vi "Module Loop.vi"(8 "error in (no error)":errorcluster, 11 "Data Processor Module in":refnum<class "Data Processor Module.lvclass">) -> (0 "error out":errorcluster, 3 "Data Processor Module out":refnum<class "Data Processor Module.lvclass">)   [LabVIEW 2020, in "VolatusData.lvlib" / "Data Processor Module.lvclass"]
uses:
  Data Processor Module.lvclass
  C:/dev/lv20CE/relink/lv-volatus/Volatus/Module/Module.lvclass
  Volatus/Module/Module.lvclass
  New Data.ctl
  Volatus/Module/Module.lvclass/Module.ctl
  <vilib>/Utility/error.llb/Error Cluster From Error Code.vi
  Data Processor Module.lvclass/Data Processor Module.ctl
  VolatusData.lvlib
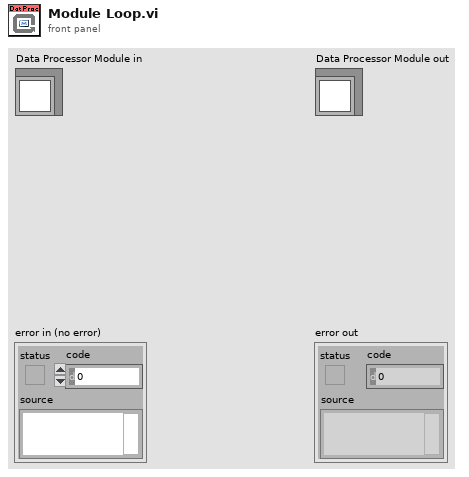
[diagram p1: front panel]
types:
  T1 = typedef "VolatusData.lvlib/New Data.ctl" = cluster{"Channels":waveform(dbl)[]}
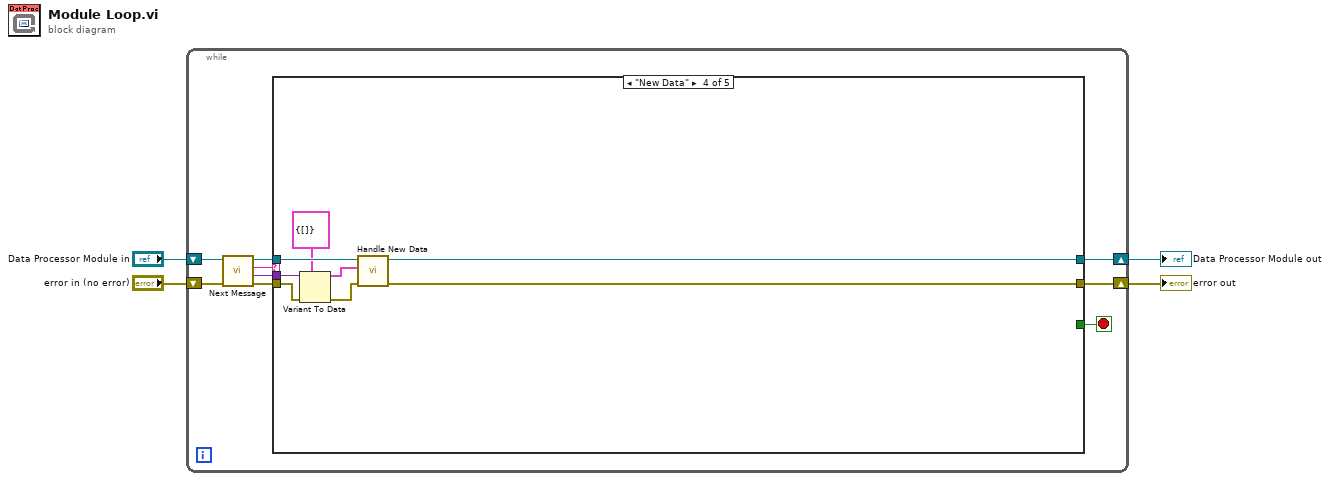
[diagram p0: block diagram]
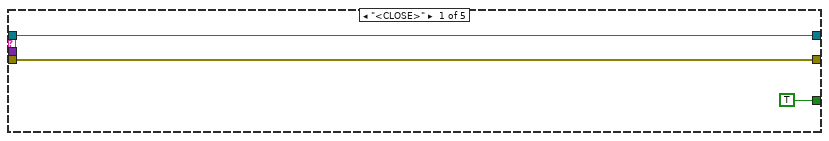
[diagram p2: hidden frame]
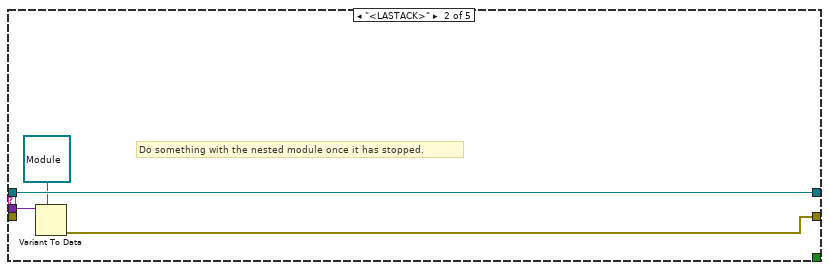
[diagram p3: hidden frame]
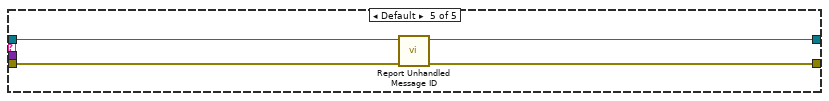
[diagram p5: hidden frame]
diagram:
  n1 = while {
    shift-right: [w8] -> w3
    shift-left: "Data Processor Module in" -> [w13]
    shift-right: [w7] -> w2
    shift-left: "error in (no error)" -> [w12]
    stop <- w6 stop-if-true
    n2 = call "Next Message.vi"("error in (no error)"=w12, "Module in"=w13) -> ("error out"=w11:errorcluster, "Data"=w5:variant, "ID"=w10:string, "Module out"=w9:refnum<class "Data Processor Module.lvclass">)  [unwired: 6 in]
    n3 = case shown="\"New Data\"" w10 {
      tunnel: w11 -> [w14 _ w21 w28 w34]
      tunnel: w9 -> [w15 w20 w22 w30 w32]
      tunnel: [w15 w20 w22 w26 w31] -> w8
      tunnel: [w14 w17 w21 w23 w33] -> w7
      tunnel: [TRUE _ _ _ _] -> w6
      tunnel: w5 -> [_ w19 _ w29 _]
      frame "<CLOSE>" {
      }
      frame "<LASTACK>" {
        # "Do something with the nested module once it has stopped."
        n4 = Variant To Data(type=refnum<class "Module.lvclass"> refnum ("Volatus:Module"), Variant=w19) -> (error out=w17:errorcluster)  [unwired: 1 in, 1 out]
      }
      frame "<TIMEOUT>" {
        # "No message for this module was received in time"
      }
      frame "New Data" {
        n5 = Variant To Data(error in=w28, type=T1 {"Channels"=[]} ("New Data"), Variant=w29) -> (data=w25:T1, error out=w24:errorcluster)
        n6 = call "Handle New Data.vi"("error in (no error)"=w24, "New Data"=w25, "Data Processor Module in"=w30) -> ("error out"=w23:errorcluster, "Data Processor Module out"=w26:refnum<class "Data Processor Module.lvclass">)  [unwired: 7 in]
      }
      frame Default {
        n7 = call "Report Unhandled Message ID.vi"("error in (no error)"=w34, "Module in"=w32) -> ("error out"=w33:errorcluster, "Module out"=w31:refnum<class "Data Processor Module.lvclass">)  [unwired: 8 in]
      }
    }
  }
  "error out" <- w2
  "Data Processor Module out" <- w3
